vi "saveTimeSeries.vi"   [LabVIEW 2011]
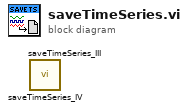
[diagram p0: block diagram]
diagram:
  n1 = call "saveTimeSeries_IV.vi"() -> ()  [unwired: 15 in, 1 out]
  n2 = call "saveTimeSeries_III.vi"() -> ()  [unwired: 15 in, 1 out]
